vi "Rule Check.vi"(8 "error in (no error)":errorcluster, 11 "Text based Communications Test in":refnum<class "Text based Communications Test.lvclass">) -> (0 "error out":errorcluster, 3 "Text based Communications Test out":refnum<class "Text based Communications Test.lvclass">)   [LabVIEW 2017, in "Text based Communications Test.lvlib" / "Text based Communications Test.lvclass"]
uses:
  Text based Communications Test.lvclass
  Text based Communications Test.lvclass/Text based Communications Test.ctl
  <vilib>/regexp/Match Regular Expression.xnode
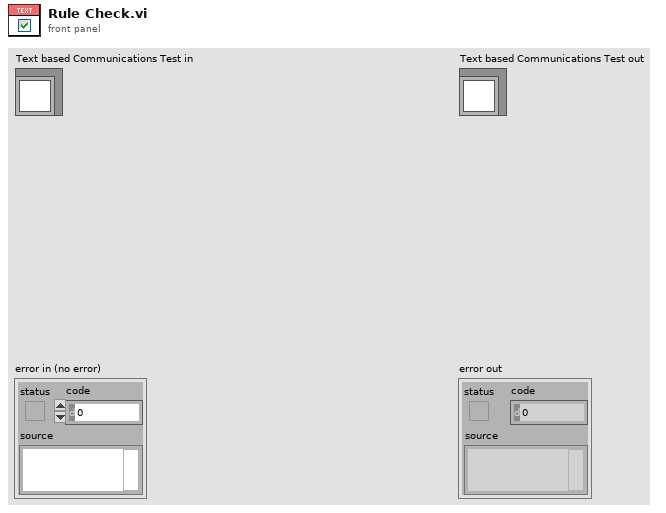
[diagram p1: front panel]
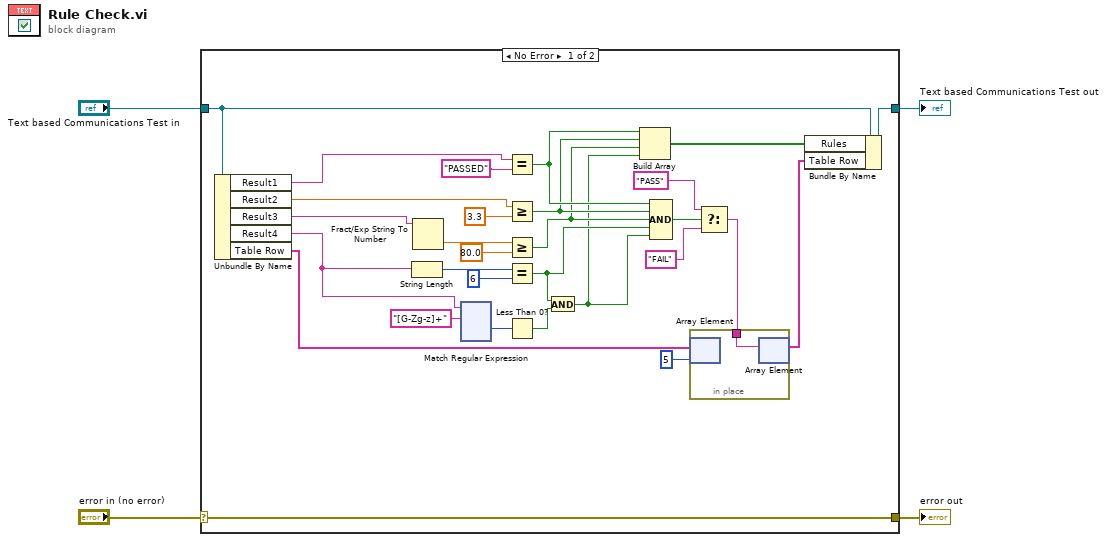
[diagram p0: block diagram]
diagram:
  n1 = case shown="No Error" "error in (no error)" {
    selector: "error in (no error)" -> [w33 w150]
    tunnel: [w33 w150] -> w3
    tunnel: [w19 w149] -> w1
    tunnel: "Text based Communications Test in" -> [w24 w149]
    frame No Error {
      n2 = Unbundle By Name(w24) -> ("Result1"=w21:string, "Result2"=w20:dbl, "Result3"=w22:string, "Result4"=w23:string, "Table Row"=w8:string[])
      n3 = String Length(string=w23) -> (length=w28:i32)
      n4 = Fract/Exp String To Number(string=w22) -> (number=w30:dbl)  [unwired: 3 in, 1 out]
      n5 = xnode "Match Regular Expression"("input string"=w23, "regular expression"="[G-Zg-z]+") -> ("offset past match"=w26:i32)  [unwired: 4 in, 4 out]
      n6 = Equal?(x=w21, y="PASSED") -> (x = y?=w17:bool)
      n7 = Greater Or Equal?(x=w20, y=3.3) -> (x >= y?=w16:bool)
      n8 = Greater Or Equal?(x=w30, y=80.0) -> (x >= y?=w15:bool)
      n9 = Equal?(x=w28, y=6) -> (x = y?=w14:bool)
      n10 = Less Than 0?(x=w26) -> (x < 0?=w18:bool)
      n11 = And(x=w14, y=w18) -> (x .and. y?=w13:bool)
      n12 = Build Array(w17, w16, w15, w13) -> (w12:bool[])
      n13 = Compound Arithmetic op=AND(w17, w16, w15, w14, w13) -> (w11:bool)
      n14 = Select(t="PASS", s=w11, f="FAIL") -> (s? t:f=w6:string)
      n15 = in-place {
        in-place-border: w6 -> [w34]
        n16 = in-place-array #1(w8, 5) -> ()  [unwired: 1 out]
        n17 = in-place-array #1(w34) -> (w5:string[])  [unwired: 1 out]
      }
      n18 = Bundle By Name(cluster=w24, "Rules"=w12, "Table Row"=w5) -> (w19:refnum<class "Text based Communications Test.lvclass">)
    }
    frame Error {
    }
  }
  "error out" <- w3
  "Text based Communications Test out" <- w1
